vi "Read Charact Standard List.vi"(8 "error in (no error)":errorcluster, 11 "Scalar Path Group in":refnum<class "Scalar Path Group.lvclass">) -> (0 "error out":errorcluster, 2 "Charact Standard List":T1[](array[typedef]), 3 "Scalar Path Group out":refnum<class "Scalar Path Group.lvclass">)   [LabVIEW 2023, in "RFFixtureCharact.Public.lvlib" / "Scalar Path Group.lvclass"]
uses:
  Scalar Path Group.lvclass
  Instruments/Cal Standard/Type Definitions/Standard Type.ctl
  Instruments/RFFixtureCharact.Instruments.lvlib
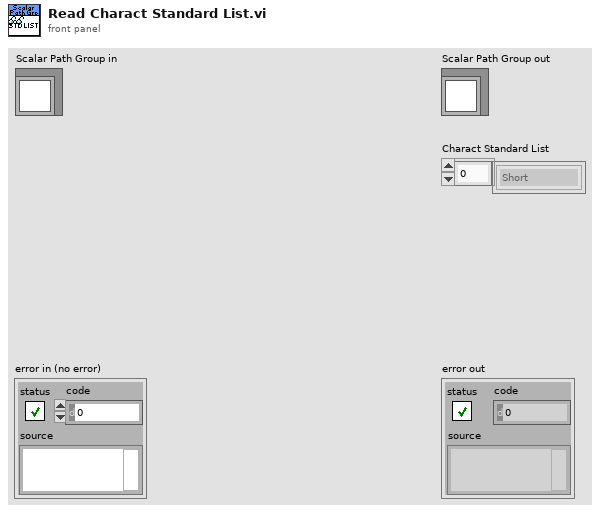
[diagram p1: front panel]
types:
  T1 = typedef "RFFixtureCharact.Instruments.lvlib/Standard Type.ctl" = enum16{"Short", "Open", "Load", "PowerMeter", "None"}
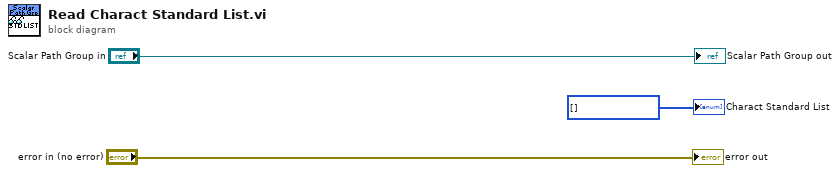
[diagram p0: block diagram]
diagram:
  w1 = T1[] [] items=["Short", "Open", "Load", "PowerMeter", "None"] ("Charact Standard List")
  "error out" <- "error in (no error)"
  "Scalar Path Group out" <- "Scalar Path Group in"
  "Charact Standard List" <- w1
